vi "Read Use Numeric Extensions.vi"(8 "error in (no error)":errorcluster, 11 "JSON Serializer in":refnum<class "JSON Serializer.lvclass">) -> (0 "error out":errorcluster, 2 "Numeric Extensions":bool, 3 "JSON Serializer out":refnum<class "JSON Serializer.lvclass">)   [LabVIEW 2013, in "JKI JSON Serialization.lvlib" / "JSON Serializer.lvclass"]
uses:
  JSON Serializer.lvclass
  JSON Serializer.lvclass/JSON Serializer.ctl
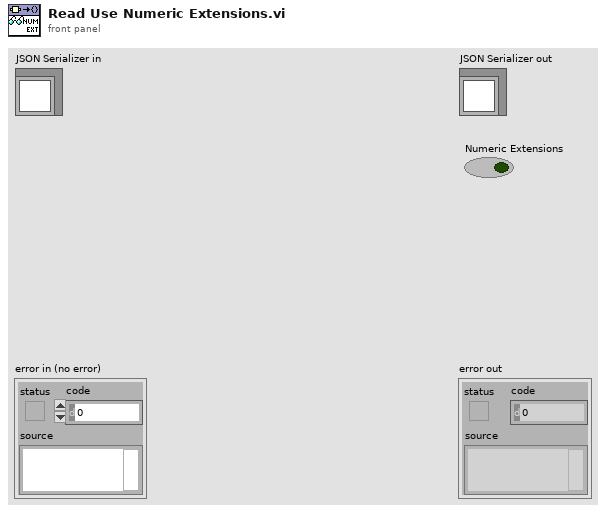
[diagram p1: front panel]
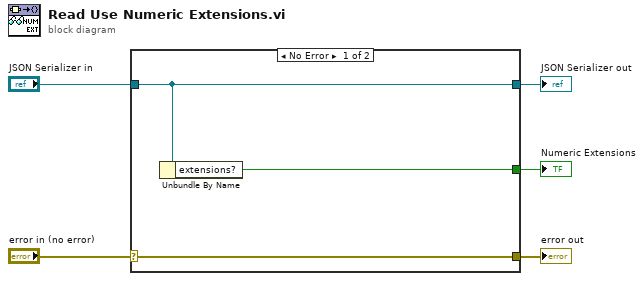
[diagram p0: block diagram]
diagram:
  n1 = case shown="No Error" "error in (no error)" {
    selector: "error in (no error)" -> [w8 w9]
    tunnel: [w8 w9] -> w4
    tunnel: [w7 w10] -> w2
    tunnel: "JSON Serializer in" -> [w7 w10]
    tunnel: [w6 _] -> w1
    frame No Error {
      n2 = Unbundle By Name(w7) -> ("extensions?"=w6:bool)
    }
    frame Error {
    }
  }
  "error out" <- w4
  "JSON Serializer out" <- w2
  "Numeric Extensions" <- w1
